vi "MISC Timestamp.vi"(8 "error in (no error)":errorcluster) -> (0 "error out":errorcluster, 3 "Timestamp":timestamp)   [LabVIEW 2017]
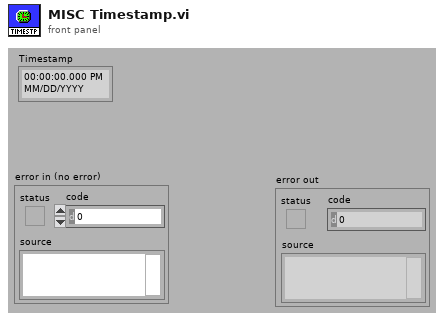
[diagram p1: front panel]
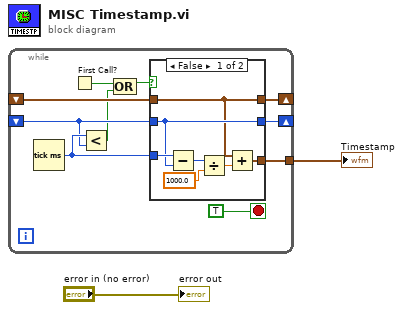
[diagram p0: block diagram]
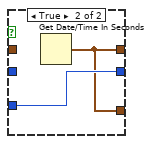
[diagram p2: hidden frame]
diagram:
  n1 = while {
    shift-right: [w10] -> _
    shift-left: _ -> [w9]
    shift-right: [w12] -> _
    shift-left: _ -> [w8]
    tunnel: [w4] -> w2
    stop <- TRUE stop-if-true
    n2 = Tick Count (ms)() -> (millisecond timer value=w11:u32)
    n3 = First Call?() -> (First Call?: T/F=w7:bool)
    n4 = Less?(x=w11, y=w8) -> (x < y?=w5:bool)
    n5 = Compound Arithmetic op=OR(w7, w5) -> (w6:bool)
    n6 = case shown="False" w6 {
      tunnel: w11 -> [w19 w21]
      tunnel: [w18 w21] -> w12
      tunnel: [w15 w20] -> w10
      tunnel: w9 -> [w15 _]
      tunnel: w8 -> [w18 _]
      tunnel: [w13 w20] -> w4
      frame False {
        n7 = Subtract(x=w19, y=w18) -> (x-y=w17:u32)
        n8 = Divide(x=w17, y=1000.0) -> (x/y=w14:dbl)
        n9 = Add(x=w15, y=w14) -> (x+y=w13:timestamp)
      }
      frame True {
        n10 = Get Date/Time In Seconds() -> (seconds since 1Jan1904=w20:timestamp)
      }
    }
  }
  "Timestamp" <- w2
  "error out" <- "error in (no error)"
